vi "Actor Core.vi"(8 "error in":errorcluster, 11 "SCADA in":refnum<class "SCADA.lvclass">) -> (0 "error out":errorcluster, 3 "Actor out":refnum<class "Actor.lvclass">)   [LabVIEW 2015, in "SCADA Core.lvlib" / "SCADA.lvclass"]
doc: "(<B>Filename</B>: Actor Framework.lvlib:Actor.lvclass:Actor Core.vi)\n\nReceives messages to the actor, reacts to them, and initiates any error handling that may shut the actor down.\n\nDescendant classes may override this VI to append parallel tasks for the actor to complete while it handles messages. Overrides use the Call Parent Method node."
uses:
  SCADA.lvclass
  <vilib>/ActorFramework/Actor/Actor.lvclass
  Logger Actor/Logger/Logger.lvclass
  SCADA.lvclass/SCADA.ctl
  Utilities/Status Messaging.llb/Status Messaging.lvlib
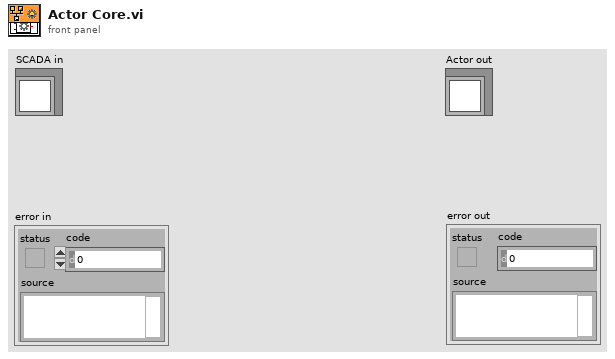
[diagram p1: front panel]
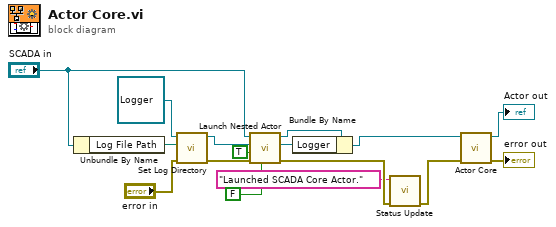
[diagram p0: block diagram]
diagram:
  n1 = Unbundle By Name("SCADA in") -> ("Log File Path"=w13:path)
  n2 = call "Set Log Directory.vi"("error in (no error)"="error in", "Log File Directory"=w13, "Logger in"=refnum<class "Logger.lvclass"> refnum ("Logger Actor.lvlib:Logger.lvclass")) -> ("error out"=w6:errorcluster, "Logger out"=w11:refnum<class "Logger.lvclass">)  [unwired: 7 in]
  n3 = call <vilib>:"Launch Nested Actor.vi"("Open Actor Core front panel? (F)"=FALSE, "error in (no error)"=w6, "Auto-stop? (T)"=TRUE, "Nested Actor"=w11, "Caller Actor in"="SCADA in") -> ("error out"=w5:errorcluster, "Nested Actor's Enqueuer"=w7:refnum<class "Message Enqueuer.lvclass">, "Caller Actor out"=w9:refnum<class "SCADA.lvclass">)  [unwired: 4 in]
  n4 = Bundle By Name(cluster=w9, "Logger"=w7) -> (w8:refnum<class "SCADA.lvclass">)
  n5 = call "Status Update.vi"("error in (no error)"=w5, "Status Update"="Launched SCADA Core Actor.") -> ("error out"=w4:errorcluster)  [unwired: 8 in, 1 out]
  n6 = call-parent "Actor Core.vi"("error in"=w4, "Actor in"=w8) -> ("error out"=→"error out":errorcluster, "Actor out"=→"Actor out":refnum<class "Actor.lvclass">)  [unwired: 8 in]
